vi "Custom Error.vi"(8 "error in (no error)":errorcluster, 11 "Custom Error":T1) -> (0 "error out":errorcluster, 3 "Classification":T2)   [LabVIEW 2019, in "Error.lvclass"]
uses:
  Error.lvclass
  <vilib>/ErrorRing/Error Ring.xnode
  <vilib>/Utility/error.llb/Error Cluster From Error Code.vi
  TypeDef/Error Classification.ctl
  TypeDef/Custom Error List.ctl
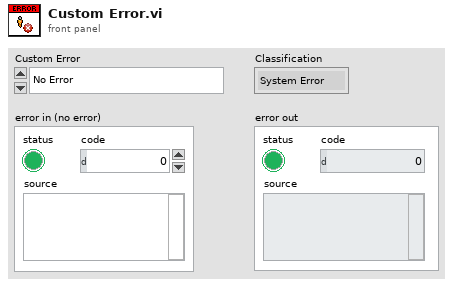
[diagram p1: front panel]
types:
  T1 = typedef "Error.lvclass/Custom Error List.ctl" = enum16{"No Error", "< --- System Errors --- >", "Lounching Modules Error", "StartApp Event Error", "Event Logging Error", "Modules Response Error", "< --- Process Errors --- >", "< --- Warnings --- >"}
  T2 = typedef "Error.lvclass/Error Classification.ctl" = enum16{"System Error", "Process Error", "Warning", "LabView built-in"}
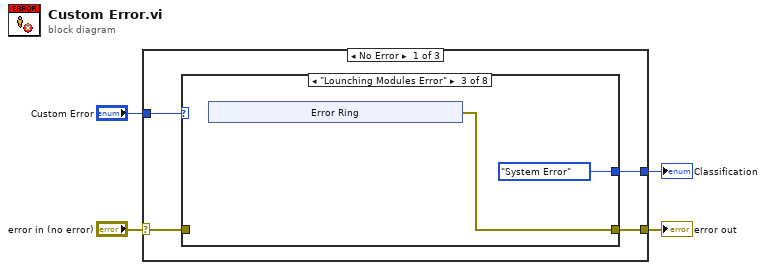
[diagram p0: block diagram]
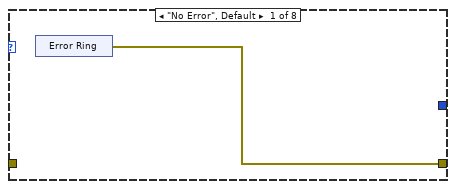
[diagram p2: hidden frame]
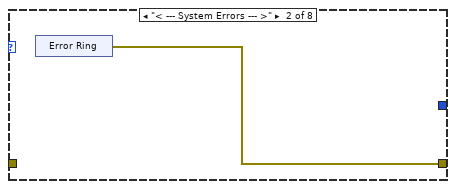
[diagram p3: hidden frame]
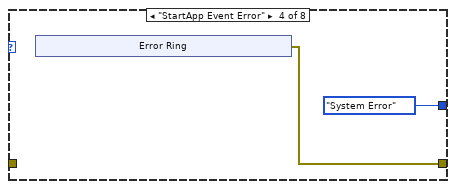
[diagram p4: hidden frame]
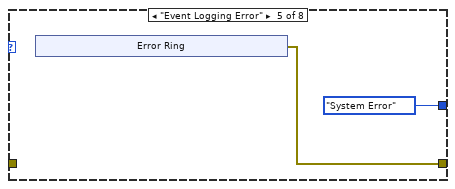
[diagram p5: hidden frame]
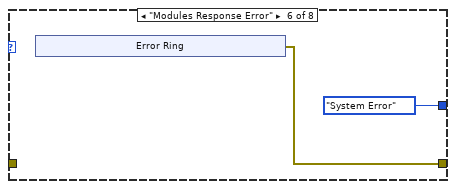
[diagram p6: hidden frame]
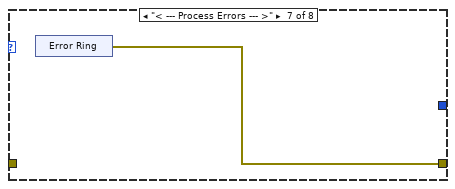
[diagram p7: hidden frame]
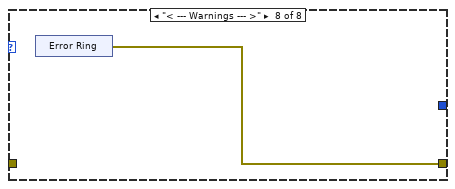
[diagram p8: hidden frame]
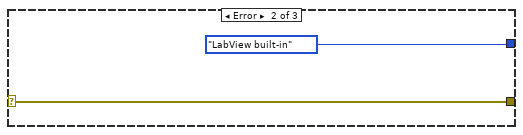
[diagram p9: hidden frame]
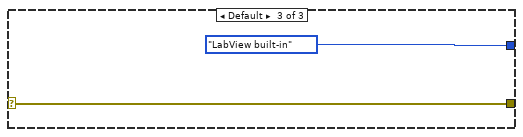
[diagram p10: hidden frame]
diagram:
  n1 = case shown="No Error" "error in (no error)" {
    selector: "error in (no error)" -> [w8 w46 w48]
    tunnel: [w7 w46 w48] -> w4
    tunnel: "Custom Error" -> [w6 _ _]
    tunnel: [w5 Error_Classification."LabView built-in" ("Classification") Error_Classification."LabView built-in" ("Classification")] -> w3
    frame No Error {
      n2 = case shown="\"Lounching Modules Error\"" w6 {
        tunnel: w8 -> [_ _ _ _ _ _ _ _]
        tunnel: [w9 w11 w14 w21 w28 w35 w41 w43] -> w7
        tunnel: [_ _ Error_Classification."System Error" ("Classification") Error_Classification."System Error" ("Classification") Error_Classification."System Error" ("Classification") Error_Classification."System Error" ("Classification") _ _] -> w5
        frame "No Error", Default {
          n3 = xnode "Error Ring"() -> ("error out"=w9:errorcluster)
        }
        frame "< --- System Errors --- >" {
          n4 = xnode "Error Ring"() -> ("error out"=w11:errorcluster)
        }
        frame "Lounching Modules Error" {
          n5 = xnode "Error Ring"() -> ("error out"=w14:errorcluster)
        }
        frame "StartApp Event Error" {
          n6 = xnode "Error Ring"() -> ("error out"=w21:errorcluster)
        }
        frame "Event Logging Error" {
          n7 = xnode "Error Ring"() -> ("error out"=w28:errorcluster)
        }
        frame "Modules Response Error" {
          n8 = xnode "Error Ring"() -> ("error out"=w35:errorcluster)
        }
        frame "< --- Process Errors --- >" {
          n9 = xnode "Error Ring"() -> ("error out"=w41:errorcluster)
        }
        frame "< --- Warnings --- >" {
          n10 = xnode "Error Ring"() -> ("error out"=w43:errorcluster)
        }
      }
    }
    frame Error {
    }
    frame Default {
    }
  }
  "error out" <- w4
  "Classification" <- w3
